vi "CHN_WND_TRC_MRKR_LMT_CHK.vi"(1 "Channel":i32=1, 2 "Window":i32=1, 3 "Trace":i32=1, 4 "Marker":i32=1, 5 "error in":errorcluster) -> (14 "error out":errorcluster, 15 "Channel":i32=1, 16 "Window":i32=1, 17 "Trace":i32=1, 18 "Marker":i32)   [LabVIEW 2018, in "PNA-X.lvlib"]
uses:
  PNA-X.lvlib
panel:
  in  "Limits":T1={"ChnMax"=16, "ChnMin"=1, "WndMax"=16, "WndMin"=1, "TrcMax"=16, "TrcMin"=1, "MarkerMax"=4, "MarkerMin"=0}
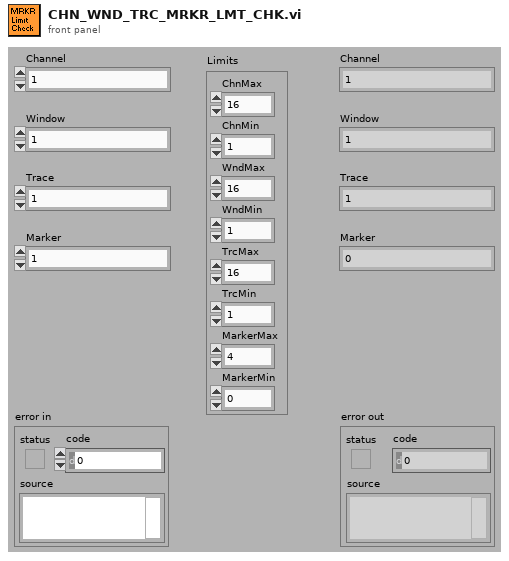
[diagram p1: front panel]
types:
  T1 = cluster{"ChnMax":i32, "ChnMin":i32, "WndMax":i32, "WndMin":i32, "TrcMax":i32, "TrcMin":i32, "MarkerMax":i32, "MarkerMin":i32}
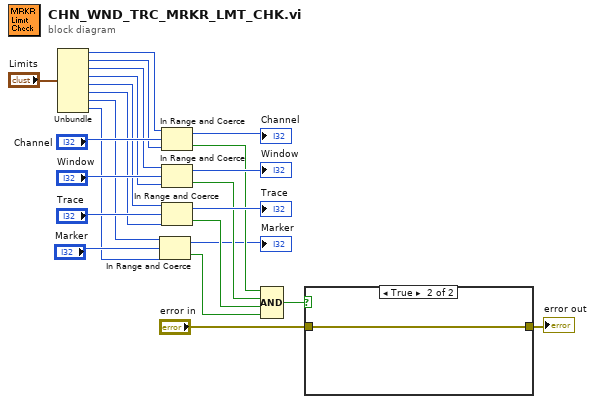
[diagram p0: block diagram]
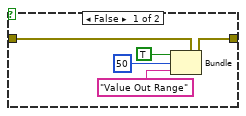
[diagram p2: hidden frame]
diagram:
  n1 = Unbundle("Limits") -> ("ChnMax"=w11:i32, "ChnMin"=w12:i32, "WndMax"=w13:i32, "WndMin"=w14:i32, "TrcMax"=w15:i32, "TrcMin"=w16:i32, "MarkerMax"=w4:i32, "MarkerMin"=w3:i32)
  n2 = In Range and Coerce(upper limit=w4, x="Marker", lower limit=w3) -> (coerced(x)=→"Marker":i32, In Range?=w1:bool)
  n3 = In Range and Coerce(upper limit=w11, x="Channel", lower limit=w12) -> (coerced(x)=→"Channel":i32, In Range?=w10:bool)
  n4 = In Range and Coerce(upper limit=w13, x="Window", lower limit=w14) -> (coerced(x)=→"Window":i32, In Range?=w9:bool)
  n5 = In Range and Coerce(upper limit=w15, x="Trace", lower limit=w16) -> (coerced(x)=→"Trace":i32, In Range?=w8:bool)
  n6 = Compound Arithmetic op=AND(w10, w9, w8, w1) -> (w7:bool)
  n7 = case shown="True" w7 {
    tunnel: "error in" -> [w28 w30]
    tunnel: [w29 w30] -> w24
    frame False {
      n8 = Bundle(cluster=w28, "status"=TRUE, "code"=50, "source"="Value Out Range") -> (w29:errorcluster)
    }
    frame True {
    }
  }
  "error out" <- w24
